vi "test.vi"() -> ()   [LabVIEW 2010]
uses:
  Tremor System v. 4.0/Classes/Timer.lvclass
panel:
  in  "reset":bool
  in  "Spin?":bool
  in  "speed":sgl=180.0
  in  "stop":bool
  out "rcos(x)":dbl
  out "rsin(x)":dbl
  in  "radius out":i16
  out "new picture":picture
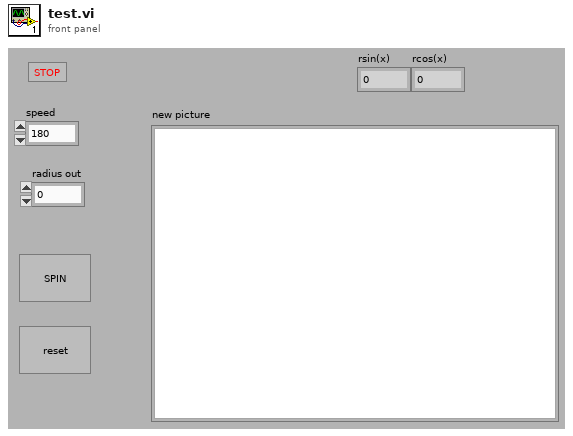
[diagram p1: front panel]
types:
  T1 = typedef "LVBoundsTypeDef.ctl" = cluster{"Width":u32, "Height":u32}
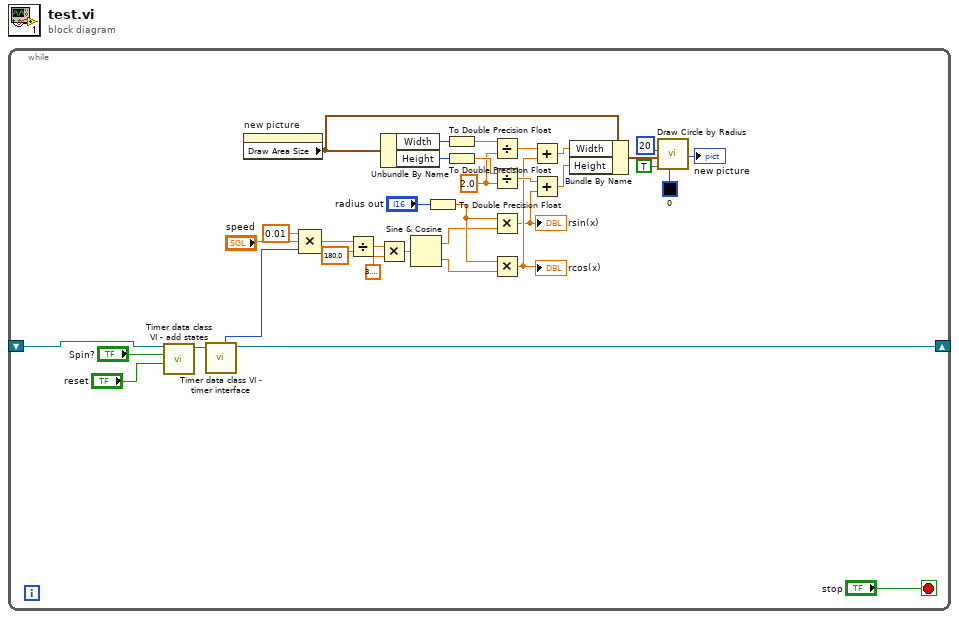
[diagram p0: block diagram]
diagram:
  n1 = while {
    shift-right: [w4] -> _
    shift-left: _ -> [w3]
    stop <- "stop" stop-if-true
    w27 = 2.0 ("radius")
    n2 = call-dynamic "Timer data class VI - add states.vi"("Reset"="reset", "Start/Stop"="Spin?", "Timer in"=w3) -> ("Timer out"=w5:refnum<class "Timer.lvclass">)  [unwired: 7 in, 1 out]
    n3 = call-dynamic "Timer data class VI - timer interface.vi"("Timer in"=w5) -> ("Timer out"=w4:refnum<class "Timer.lvclass">, "Milliseconds"=w1:u32)  [unwired: 6 in, 3 out]
    n4 = property on="new picture" class="Pict"() -> ("Draw Area Size"=w31:T1)  [unwired: 2 in, 2 out]
    n5 = Compound Arithmetic op=MULTIPLY(0.01, "speed", w1) -> (w9:dbl)
    n6 = Divide(x=w9, y=180.0) -> (x/y=w21:dbl)
    n7 = Multiply(x=w21, y=3.141592653589793) -> (x*y=w19:dbl)
    n8 = Unbundle By Name(w31) -> ("Width"=w33:u32, "Height"=w32:u32)
    n9 = Sine & Cosine(0:w19) -> (1:w24:dbl, 2:w23:dbl)
    n10 = To Double Precision Float(number="radius out") -> (double precision float=w25:dbl)
    n11 = To Double Precision Float(number=w33) -> (double precision float=w29:dbl)
    n12 = To Double Precision Float(number=w32) -> (double precision float=w28:dbl)
    n13 = Divide(x=w29, y=w27) -> (x/y=w17:dbl)
    n14 = Divide(x=w28, y=w27) -> (x/y=w18:dbl)
    n15 = Multiply(x=w25, y=w24) -> (x*y=w15:dbl)
    "rsin(x)" <- w15
    n16 = Multiply(x=w25, y=w23) -> (x*y=w16:dbl)
    "rcos(x)" <- w16
    n17 = Add(x=w17, y=w16) -> (x+y=w13:dbl)
    n18 = Add(x=w18, y=w15) -> (x+y=w14:dbl)
    n19 = Bundle By Name(cluster=w31, "Width"=w13, "Height"=w14) -> (w30:T1)
    n20 = call <vilib>:"Draw Circle by Radius.vi"("color(black)"=u32 0, "fill?(F)"=TRUE, "pixel center"=w30, "radius"=i16 20) -> ("new picture"=→"new picture":picture)  [unwired: 7 in]
  }
